vi "Image2WallDistances2.vi"(3 "error in (no error)":errorcluster, 5 "Image Src":T3) -> (0 "error out":errorcluster, 2 "Walls":T1(array[cluster]))   [LabVIEW 2009, in "ImageAnalysis.lvlib"]
uses:
  ImageAnalysis.lvlib
  <vilib>/vision/Image Controls.llb/IMAQ Image.ctl
  <vilib>/vision/Shape Detection.llb/ShapeDetectionMatchOptions.ctl
  <vilib>/vision/Pattern Matching.llb/IMAQ Match Range Setting.ctl
  <vilib>/vision/NI_Vision_Development_Module.lvlib
  ImageProcessing.lvlib
panel:
  in  "Wall":T2
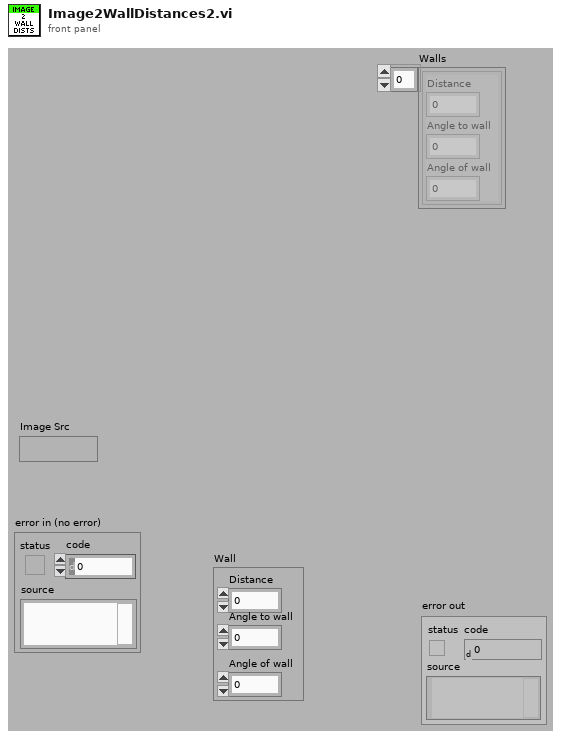
[diagram p1: front panel]
types:
  T1 = cluster{"Distance":dbl, "Angle to wall":dbl, "Angle of wall":dbl}[]
  T2 = cluster{"Distance":dbl, "Angle to wall":dbl, "Angle of wall":dbl}
  T3 = typedef "IMAQ Image.ctl" = refnum<image>
  T4 = typedef "ShapeDetectionMatchOptions.ctl" = cluster{"Rotation":bool, "Scale":bool, "Occlusion":bool, "Range Settings":T5[]}
  T5 = typedef "IMAQ Match Range Setting.ctl" = cluster{"Match Constraints":u32, "Min":dbl, "Max":dbl}
  T6 = cluster{"Min Major Radius":dbl, "Max Major Radius":dbl, "Min Minor Radius":dbl, "Max Minor Radius":dbl}
  T7 = cluster{"Position":cluster{"X":sgl, "Y":sgl}, "Angle":dbl, "Major Radius":dbl, "Minor Radius":dbl, "Score":dbl}[]
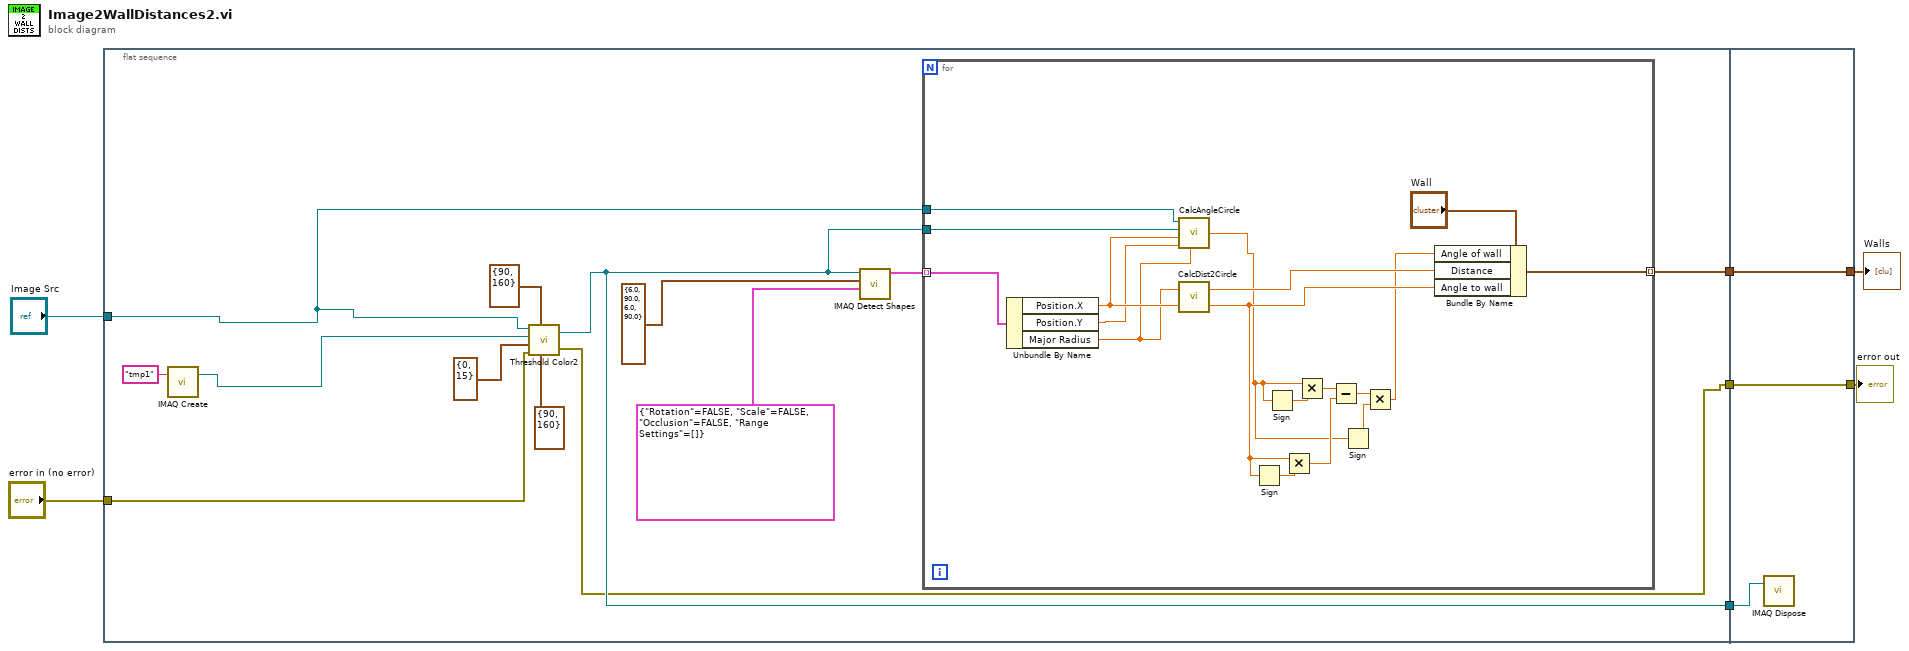
[diagram p0: block diagram]
diagram:
  n1 = flat-sequence {
    tunnel: "Image Src" -> [w12]
    tunnel: "error in (no error)" -> [w13]
    tunnel: [w16] -> w5
    tunnel: [w18] -> w3
    tunnel: [w17] -> w2
    tunnel: w5 -> [w41]
    tunnel: [w41] -> w4
    tunnel: [w40] -> w1
    tunnel: w3 -> [w40]
    tunnel: w2 -> [w39]
    frame #0 {
      n2 = call "IMAQ Create"("Image Name"="tmp1") -> ("New Image"=w11:T3)  [unwired: 4 in, 1 out]
      n3 = call "Threshold Color2.vi"("Val or Inten Range"=cluster{"Lower value":i32, "Upper value":i32} {"Lower value"=90, "Upper value"=160}, "Sat Range"=cluster{"Lower value":i32, "Upper value":i32} {"Lower value"=90, "Upper value"=160}, "error in (no error)"=w13, "Hue Range"=cluster{"Lower value":i32, "Upper value":i32} {"Lower value"=0, "Upper value"=15}, "Image Dst"=w11, "Image Src"=w12) -> ("error out"=w16:errorcluster, "Image Dst Out"=w17:T3)
      n4 = call-poly "IMAQ Detect Shapes"("Match Options"=T4 {"Rotation"=FALSE, "Scale"=FALSE, "Occlusion"=FALSE, "Range Settings"=[]}, "Ellipse Descriptor"=T6 {"Min Major Radius"=6.0, "Max Major Radius"=90.0, "Min Minor Radius"=6.0, "Max Minor Radius"=90.0}, "Image"=w17) -> ("Ellipses"=w19:T7)  [unwired: 6 in, 2 out]
      n5 = for {
        tunnel: w19 -> [w38] mode=indexing
        tunnel: w17 -> [w37]
        tunnel: w12 -> [w33]
        tunnel: [w30] -> w18 mode=indexing
        n6 = Unbundle By Name(w38) -> ("Position.X"=w36:sgl, "Position.Y"=w35:sgl, "Major Radius"=w34:dbl)
        n7 = call "CalcAngleCircle.vi"("Original Image"=w33, "Filtered Image"=w37, "X Coordinate"=w36, "Y Coordinate"=w35, "Vertical radius"=w34) -> ("Angle in rad"=w22:dbl)
        n8 = call "CalcDist2Circle.vi"("X-cords"=w36, "Height of circle"=w34) -> ("Angle to circle"=w27:dbl, "Distance"=w31:dbl)
        n9 = Sign(1:w27) -> (0:w28:dbl)
        n10 = Sign(1:w22) -> (0:w29:dbl)
        n11 = Multiply(x=w27, y=w28) -> (x*y=w25:dbl)
        n12 = Multiply(x=w22, y=w29) -> (x*y=w26:dbl)
        n13 = Subtract(x=w26, y=w25) -> (x-y=w24:dbl)
        n14 = Sign(1:w22) -> (0:w23:dbl)
        n15 = Multiply(x=w24, y=w23) -> (x*y=w21:dbl)
        n16 = Bundle By Name(cluster="Wall", "Angle of wall"=w21, "Distance"=w31, "Angle to wall"=w27) -> (w30:T2)
      }
    }
    frame #1 {
      n17 = call "IMAQ Dispose"("Image"=w39) -> ()  [unwired: 5 in, 1 out]
    }
  }
  "error out" <- w4
  "Walls" <- w1
